vi "TagMetadataToImage.vi"(8 "error in (no error)":errorcluster, 10 "Image In":T1, 11 "DAQ_QPT_Throlab in":refnum<class "DAQ_QPT_Throlab.lvclass">) -> (0 "error out":errorcluster, 2 "Image Out":T1, 3 "DAQ_QPT_Throlab out":refnum<class "DAQ_QPT_Throlab.lvclass">)   [LabVIEW 2020, in "DAQ_QPT_Throlab.lvlib" / "DAQ_QPT_Throlab.lvclass"]
uses:
  DAQ_QPT_Throlab.lvclass
  <vilib>/vision/Image Controls.llb/IMAQ Image.ctl
  DAQ_QPT_Throlab.lvclass/DAQ_QPT_Throlab.ctl
  Hardware Abstraction Layer/Component/DAQ/DAQ/DAQ.lvclass
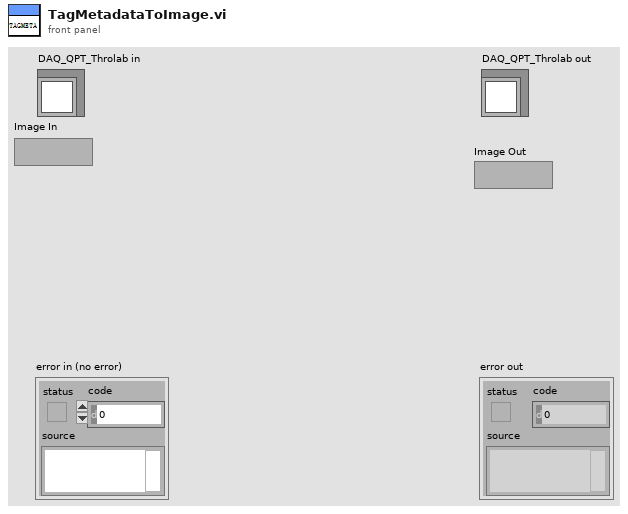
[diagram p1: front panel]
types:
  T1 = typedef "IMAQ Image.ctl" = refnum<image>
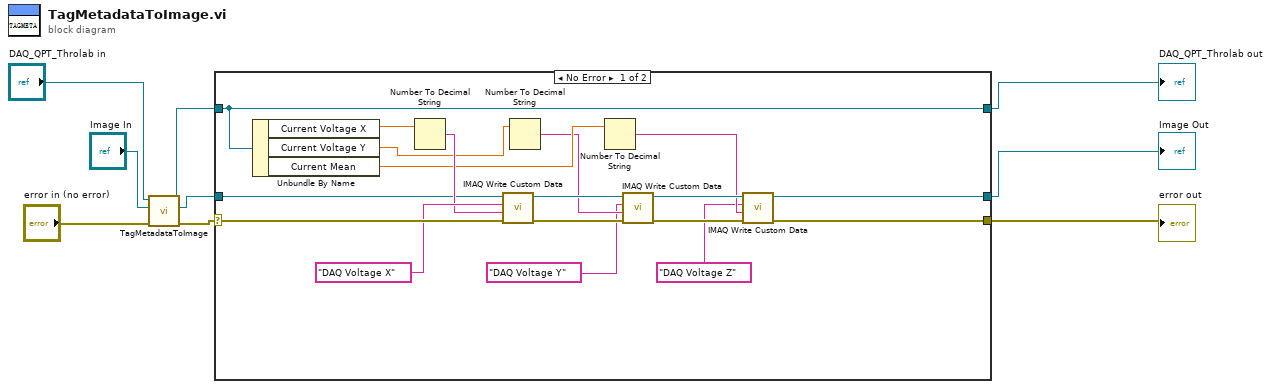
[diagram p0: block diagram]
diagram:
  n1 = call-parent "TagMetadataToImage.vi"("error in (no error)"="error in (no error)", "Image In"="Image In", "Device in"="DAQ_QPT_Throlab in") -> ("error out"=w6:errorcluster, "Image Out"=w5:T1, "Device out"=w4:refnum<class "DAQ_QPT_Throlab.lvclass">)  [unwired: 6 in]
  n2 = case shown="No Error" w6 {
    selector: w6 -> [w25 w30]
    tunnel: [w20 w30] -> w1
    tunnel: w5 -> [w21 w29]
    tunnel: [w19 w29] -> w2
    tunnel: [w27 w28] -> w3
    tunnel: w4 -> [w27 w28]
    frame No Error {
      n3 = Unbundle By Name(w27) -> ("Current Voltage X"=w26:dbl, "Current Voltage Y"=w15:dbl, "Current Mean"=w14:dbl)
      n4 = Number To Decimal String(number=w26) -> (decimal integer string=w22:string)  [unwired: 1 in]
      n5 = call "IMAQ Write Custom Data"("error in (no error)"=w25, "Custom Data In"=w22, "Key"="DAQ Voltage X", "Image"=w21) -> ("error out"=w24:errorcluster, "Image Out"=w17:T1)  [unwired: 6 in]
      n6 = Number To Decimal String(number=w15) -> (decimal integer string=w12:string)  [unwired: 1 in]
      n7 = Number To Decimal String(number=w14) -> (decimal integer string=w13:string)  [unwired: 1 in]
      n8 = call "IMAQ Write Custom Data"("error in (no error)"=w24, "Custom Data In"=w12, "Key"="DAQ Voltage Y", "Image"=w17) -> ("error out"=w18:errorcluster, "Image Out"=w16:T1)  [unwired: 6 in]
      n9 = call "IMAQ Write Custom Data"("error in (no error)"=w18, "Custom Data In"=w13, "Key"="DAQ Voltage Z", "Image"=w16) -> ("error out"=w20:errorcluster, "Image Out"=w19:T1)  [unwired: 6 in]
    }
    frame Error {
    }
  }
  "error out" <- w1
  "DAQ_QPT_Throlab out" <- w3
  "Image Out" <- w2
